vi "Build Endpoint.vi"(8 "error in (no error)":errorcluster, 9 "Port":u16, 10 "Address":string, 11 "RemoteControl.STM in":refnum<class "RemoteControl.STM.lvclass">) -> (0 "error out":errorcluster, 3 "RemoteControl.STM out":refnum<class "RemoteControl.STM.lvclass">)   [LabVIEW 2020, in "RemoteControl.STM.lvclass"]
uses:
  RemoteControl.STM.lvclass
  RemoteControl/RemoteControl.lvclass
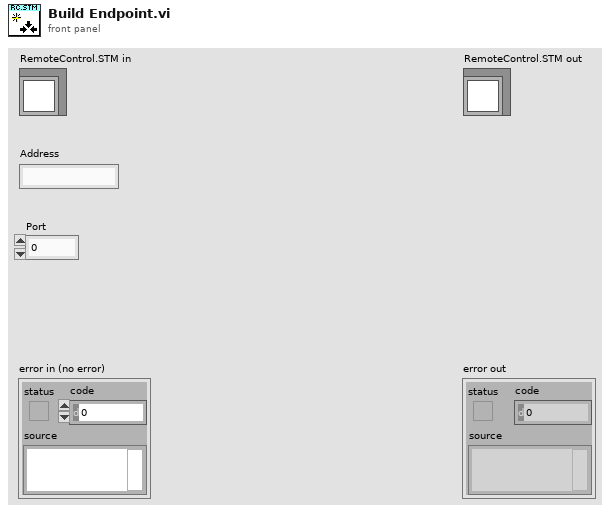
[diagram p1: front panel]
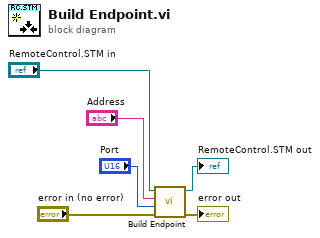
[diagram p0: block diagram]
diagram:
  n1 = call-parent "Build Endpoint.vi"("error in (no error)"="error in (no error)", "Port"="Port", "Address"="Address", "RemoteControl in"="RemoteControl.STM in") -> ("error out"=→"error out":errorcluster, "RemoteControl out"=→"RemoteControl.STM out":refnum<class "RemoteControl.STM.lvclass">)  [unwired: 6 in]
